vi "open or close panel.vi"(8 "error in (no error)":errorcluster caption="错误输入（无错误）", 10 "布尔":bool, 11 "前面板控制 输入":refnum<class "前面板控制.lvclass">) -> (0 "error out":errorcluster caption="错误输出", 3 "前面板控制 输出":refnum<class "前面板控制.lvclass">)   [LabVIEW 2015, in "前面板控制.lvlib" / "前面板控制.lvclass"]
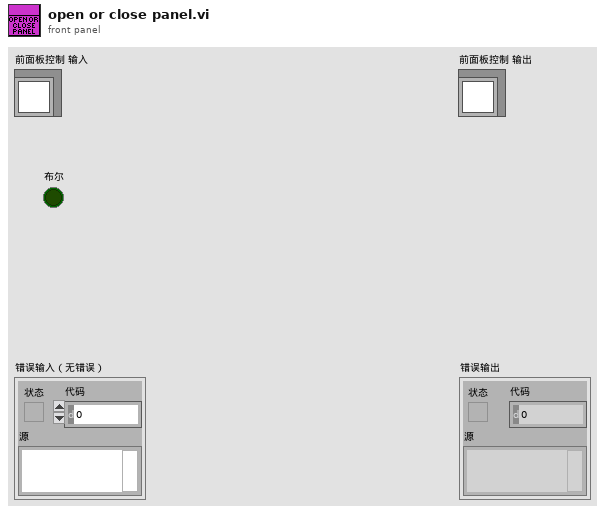
[diagram p1: front panel]
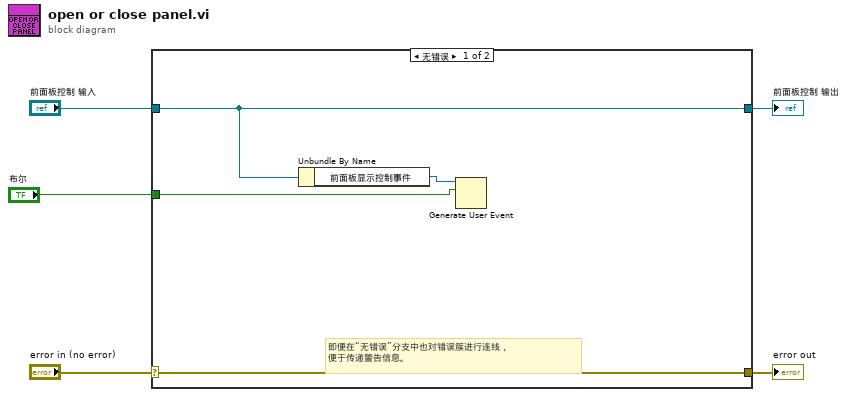
[diagram p0: block diagram]
diagram:
  n1 = case shown="无错误" "error in (no error)" {
    selector: "error in (no error)" -> [w9 w11]
    tunnel: [w9 w11] -> w4
    tunnel: [w8 w10] -> w2
    tunnel: "前面板控制 输入" -> [w8 w10]
    tunnel: "布尔" -> [w6 _]
    frame No Error {
      # "即便在“无错误”分支中也对错误簇进行连线，\n便于传递警告信息。"
      n2 = Unbundle By Name(w8) -> ("前面板显示控制事件"=w7:refnum<user-event>)
      n3 = Generate User Event(user event=w7, event data cluster=w6) -> ()  [unwired: 2 in, 2 out]
    }
    frame Error {
    }
  }
  "error out" <- w4
  "前面板控制 输出" <- w2
